vi "Constants.vi"() -> ()   [LabVIEW 2017, in "Waveform-Processing-Custom-Device Shared.lvlib"]
doc: "Use this Global VI to access the GUIDs assigned to the page resources of the Custom Device.\nThis Contains the GUID's"
uses:
  Waveform-Processing-Custom-Device Shared.lvlib
panel:
  in  "Tab Control":enum32{"GUIDS", "Constants", "Properties"}(tab)=enum."Properties"
  in  "DAQ Analog Input GUID":string="5C66C5ED-AAF0-446D-B23E-317FB174858C"
  in  "Waveform-Processing-Custom-Device Disabled":string="7b547a45-b3bf-4a70-a525-6bc55fa12b7c"
  in  "Waveform Results Section GUID":string="e38e89f1-3d1b-4012-b75e-d54b3a46b12e"
  in  "Running Average Settings GUID":string="98bae003-a8c4-4cad-9e5d-6f3690f27bc7"
  in  "Waveform-Processing-Custom-Device":string="2e5751d4-f26f-4961-8df7-f46ae00d1276"
  in  "Min SP Results Channel Group":string="MINSPResultsChannelGroup"
  in  "Max SP Results Channel Group":string="MAXSPResultsChannelGroup"
  in  "Running Average Parameters Channel Group":string="Running Average Parameters Channel Group"
  in  "Single Point Result Channel Group":string="Single Point Result Channel Group"
  in  "Running Average Result Channel Group":string="Running Average Result Channel Group"
  in  "Waveform Processing Custom Device Name":string="Waveform Processing Custom Device"
  in  "Running Average Period":string="Running Average Period"
  in  "Result.Section.Min.SP.Channel":string="ResultSectionMIN"
  in  "Result.Section.Max.SP.Channel":string="ResultScetionMAX"
  in  "CD.NumDAQChannels":string="NumDAQChannels"
  in  "CD.TaskRate":string="TaskRate"
  in  "CD.BufferSamples":string="BufferSamples"
  in  "CD.TaskDependencyRef":string="TaskDependencyRef"
  in  "CD.BufferSeconds":string="BufferSeconds"
  in  "CD.SelectedWaveforms":string="SelectedWfms"
  in  "CD.AvailableWfms":string="AvailableWfms"
  in  "Result.Section.Single.Point.Channel":string="ResultSinglePoint"
  in  "Running.Average.Settings.Period.Channel":string="Running_Average_Settings_Period_Channel"
  in  "Result.Section.Running.Average.Channel":string="ResultRunningAverage"
  in  "Compiled.Settings":string="CompiledSettings"
  in  "Result.Section.Wfm.Dependency":string="WfmDependency"
  in  "CD.TaskDependency":string="TaskDependency"
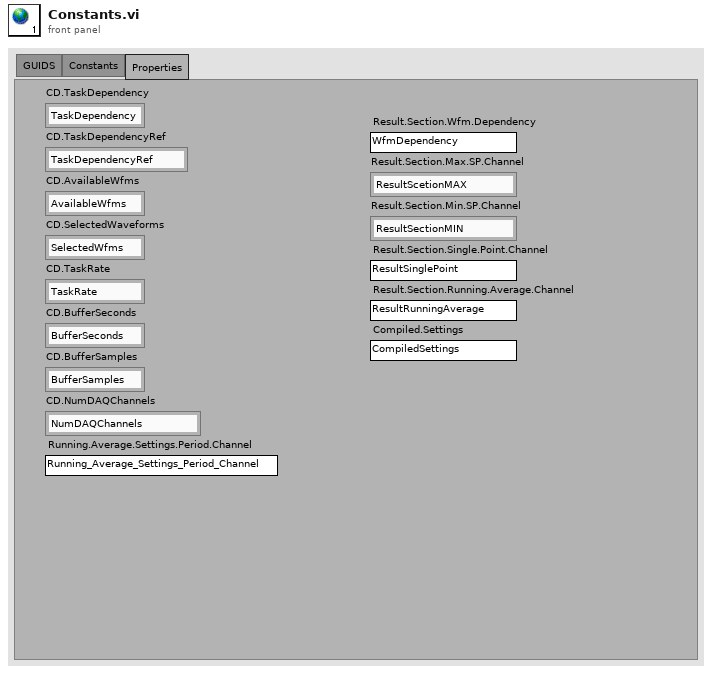
[diagram p1: front panel]
diagram:
